vi "HGF_IMAQDevice.appendData2Variant.vi"(0 "initData":variant, 1 "cameraName":string, 2 "controlMode":T2, 3 "videoMode":i32, 5 "error in (no error)":errorcluster, 7 "imageType":T1 items=["Grayscale (U8)", "Grayscale (I16)", "Grayscale (SGL)", "Complex (CSG)", "RGB (U32)", "HSL (U32)", "RGB (U64)", "Grayscale (U16)"]) -> (14 "dup initData":variant, 19 "error out":errorcluster)   [LabVIEW 2014, in "HGF_IMAQ.lvlib" / "HGF_IMAQDevice.lvclass"]
uses:
  HGF_IMAQDevice.lvclass
  Control Mode.ctl
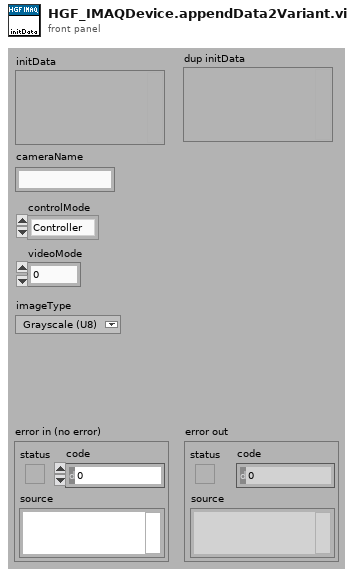
[diagram p1: front panel]
types:
  T1 = typedef "Image Type" = u32
  T2 = typedef "HGF_IMAQ.lvlib/HGF_IMAQDevice.lvclass/Control Mode.ctl" = enum16{"Controller", "Listener"}
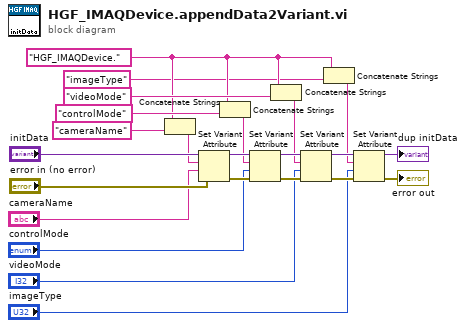
[diagram p0: block diagram]
diagram:
  w6 = "HGF_IMAQDevice." ("name")
  n1 = Concatenate Strings(w6, "cameraName" ("name")) -> (w16:string)
  n2 = Set Variant Attribute(Variant="initData", name=w16, value="cameraName", error in="error in (no error)") -> (Variant out=w20:variant, error out=w19:errorcluster)  [unwired: 1 out]
  n3 = Concatenate Strings(w6, "controlMode" ("name")) -> (w14:string)
  n4 = Set Variant Attribute(Variant=w20, name=w14, value="controlMode", error in=w19) -> (Variant out=w13:variant, error out=w12:errorcluster)  [unwired: 1 out]
  n5 = Concatenate Strings(w6, "videoMode" ("name")) -> (w7:string)
  n6 = Set Variant Attribute(Variant=w13, name=w7, value="videoMode", error in=w12) -> (Variant out=w8:variant, error out=w9:errorcluster)  [unwired: 1 out]
  n7 = Concatenate Strings(w6, "imageType" ("name")) -> (w4:string)
  n8 = Set Variant Attribute(Variant=w8, name=w4, value="imageType", error in=w9) -> (Variant out=→"dup initData":variant, error out=→"error out":errorcluster)  [unwired: 1 out]
